vi "Untitled 1.vi"() -> ()   [LabVIEW 2022 SP3]
uses:
  <vilib>/Instr/_visa.llb/VISA Configure Serial Port (Instr).vi
panel:
  out "Boolean 2":bool
  out "value 4":dbl
  out "value 3":dbl
  out "value 2":dbl
  out "value":dbl
  in  "VISA resource name":refnum<visa-resource-name>
  out "Boolean":bool
  in  "stop":bool
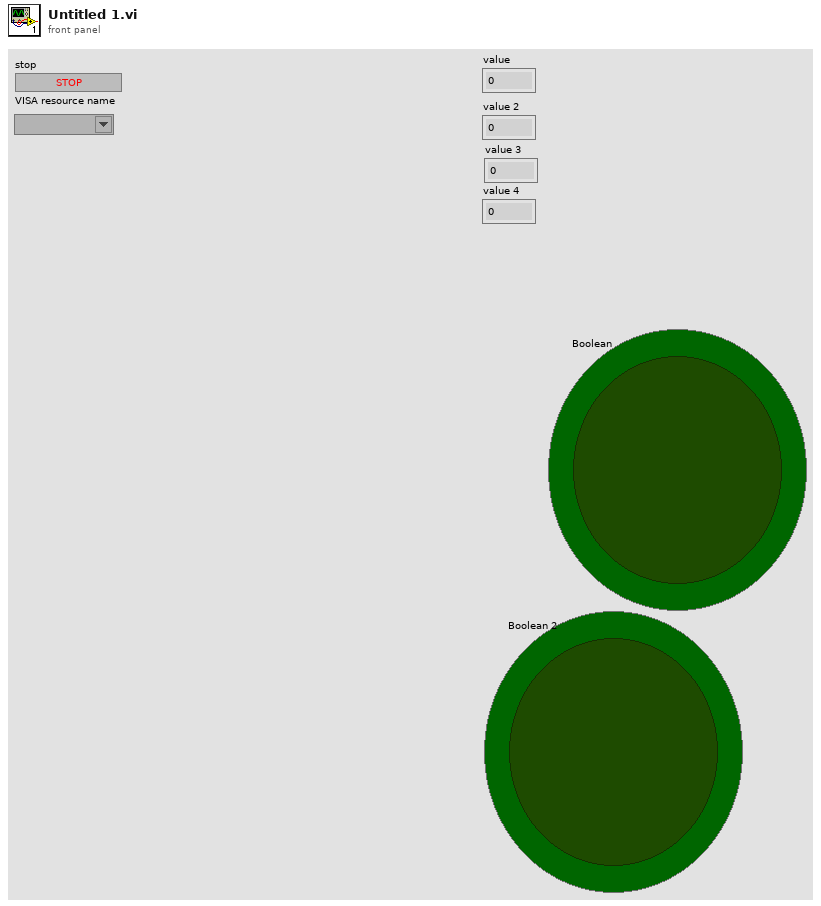
[diagram p1: front panel]
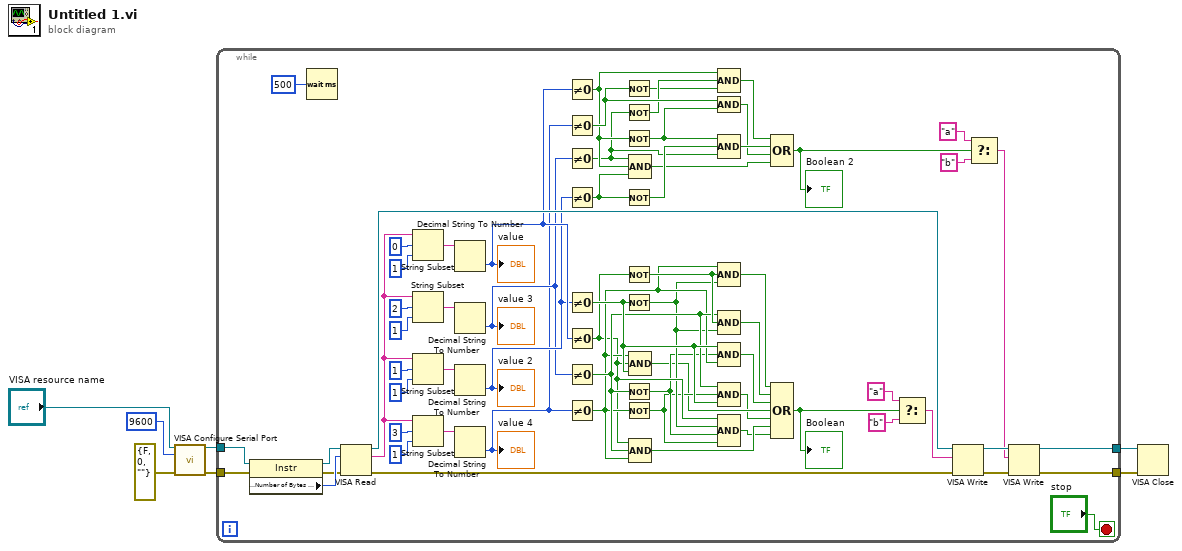
[diagram p0: block diagram]
diagram:
  n1 = call-poly "VISA Configure Serial Port"("VISA resource name"="VISA resource name", "baud rate (9600)"=u32 9600, "error in (no error)"=errorcluster {"status"=FALSE, "code"=0, "source"=""}) -> ("VISA resource name out"=w4:refnum<visa-resource-name>, "error out"=w3:errorcluster)  [unwired: 11 in]
  n2 = while {
    tunnel: w4 -> [w68]
    tunnel: w3 -> [w66]
    tunnel: [w42] -> w2
    tunnel: [w41] -> w1
    stop <- "stop" stop-if-true
    n3 = property class="Instr"(reference=w68, error in=w66) -> (reference out=w67:refnum<visa-resource-name>, error out=w65:errorcluster, "Serial Settings:Number of Bytes at Serial Port"=w69:u32)
    n4 = Wait (ms)(milliseconds to wait=u32 500) -> ()  [unwired: 1 out]
    n5 = VISA Read(VISA resource name=w67, byte count=w69, error in (no error)=w65) -> (VISA resource name out=w50:refnum<visa-resource-name>, read buffer=w56:string, error out=w49:errorcluster)  [unwired: 1 out]
    n6 = String Subset(string=w56, offset (0)=0, length (rest)=1 ("length (rest)")) -> (substring=w63:string)
    n7 = String Subset(string=w56, offset (0)=2, length (rest)=1 ("length (rest)")) -> (substring=w54:string)
    n8 = String Subset(string=w56, offset (0)=1, length (rest)=1 ("length (rest)")) -> (substring=w55:string)
    n9 = String Subset(string=w56, offset (0)=3, length (rest)=1 ("length (rest)")) -> (substring=w53:string)
    n10 = Decimal String To Number(string=w63) -> (number=w24:i32)  [unwired: 2 in, 1 out]
    "value" <- w24
    n11 = Decimal String To Number(string=w54) -> (number=w22:i32)  [unwired: 2 in, 1 out]
    "value 3" <- w22
    n12 = Decimal String To Number(string=w55) -> (number=w23:i32)  [unwired: 2 in, 1 out]
    "value 2" <- w23
    n13 = Decimal String To Number(string=w53) -> (number=w21:i32)  [unwired: 2 in, 1 out]
    "value 4" <- w21
    n14 = Not Equal To 0?(x=w24) -> (x != 0?=w16:bool)
    n15 = Not Equal To 0?(x=w21) -> (x != 0?=w18:bool)
    n16 = Not Equal To 0?(x=w22) -> (x != 0?=w8:bool)
    n17 = Not Equal To 0?(x=w23) -> (x != 0?=w17:bool)
    n18 = Not Equal To 0?(x=w23) -> (x != 0?=w39:bool)
    n19 = Not Equal To 0?(x=w24) -> (x != 0?=w36:bool)
    n20 = Not Equal To 0?(x=w22) -> (x != 0?=w38:bool)
    n21 = Not Equal To 0?(x=w21) -> (x != 0?=w37:bool)
    n22 = Not(x=w18) -> (.not. x?=w14:bool)
    n23 = Not(x=w8) -> (.not. x?=w15:bool)
    n24 = Not(x=w16) -> (.not. x?=w20:bool)
    n25 = Not(x=w17) -> (.not. x?=w19:bool)
    n26 = Not(x=w36) -> (.not. x?=w40:bool)
    n27 = Not(x=w39) -> (.not. x?=w35:bool)
    n28 = Not(x=w38) -> (.not. x?=w34:bool)
    n29 = Not(x=w37) -> (.not. x?=w33:bool)
    n30 = Compound Arithmetic op=AND(w8, w16, w17) -> (w10:bool)
    n31 = Compound Arithmetic op=AND(w37, w36, w39) -> (w29:bool)
    n32 = Compound Arithmetic op=AND(w36, w38, w37) -> (w27:bool)
    n33 = Compound Arithmetic op=AND(w16, w15, w14) -> (w13:bool)
    n34 = Compound Arithmetic op=AND(w18, w20) -> (w11:bool)
    n35 = Compound Arithmetic op=AND(w20, w19, w8) -> (w12:bool)
    n36 = Compound Arithmetic op=AND(w37, w40, w35) -> (w32:bool)
    n37 = Compound Arithmetic op=AND(w38, w40, w35) -> (w31:bool)
    n38 = Compound Arithmetic op=AND(w39, w34, w37) -> (w30:bool)
    n39 = Compound Arithmetic op=AND(w38, w33, w39) -> (w28:bool)
    n40 = Compound Arithmetic op=AND(w36, w35, w34, w33) -> (w26:bool)
    n41 = Compound Arithmetic op=OR(w13, w12, w11, w10) -> (w9:bool)
    "Boolean 2" <- w9
    n42 = Compound Arithmetic op=OR(w32, w31, w30, w29, w28, w27, w26) -> (w25:bool)
    "Boolean" <- w25
    n43 = Select(t="a", s=w25, f="b") -> (s? t:f=w48:string)
    n44 = VISA Write(VISA resource name=w50, write buffer=w48, error in (no error)=w49) -> (VISA resource name out=w45:refnum<visa-resource-name>, error out=w43:errorcluster)  [unwired: 1 out]
    n45 = Select(t="a", s=w9, f="b") -> (s? t:f=w44:string)
    n46 = VISA Write(VISA resource name=w45, write buffer=w44, error in (no error)=w43) -> (VISA resource name out=w42:refnum<visa-resource-name>, error out=w41:errorcluster)  [unwired: 1 out]
  }
  n47 = VISA Close(VISA resource name=w2, error in (no error)=w1) -> ()  [unwired: 1 out]
